vi "TL_Dt.vi"(2 "Dt (s)":i32, 3 "t0":dbl) -> (0 "Gauge":dbl, 1 "STOP":bool)   [LabVIEW 2015]
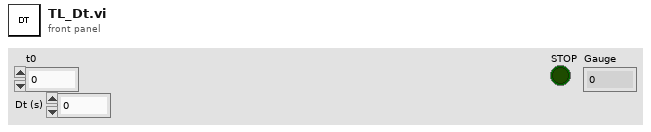
[diagram p1: front panel]
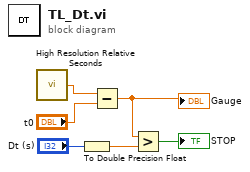
[diagram p0: block diagram]
diagram:
  n1 = call <vilib>:"High Resolution Relative Seconds.vi"() -> ("relative seconds"=w6:dbl)
  n2 = To Double Precision Float(number="Dt (s)") -> (double precision float=w1:dbl)
  n3 = Subtract(x=w6, y="t0") -> (x-y=w3:dbl)
  "Gauge" <- w3
  n4 = Greater?(x=w3, y=w1) -> (0:→"STOP":bool)
